vi "OP Model.vi"(8 "error in (no error)":errorcluster, 9 "Enum":enum16{"init", "Read", "Write"}(ring)=enum."Read", 10 "ArrayStr":string[](array[string]), 11 "Path":path) -> (0 "error out":errorcluster, 2 "ArrayStr out":string[](array[string]), 3 "Path out":path)   [LabVIEW 2014]
uses:
  <vilib>/Utility/xml.llb/Read From XML File(string).vi
  <vilib>/Utility/xml.llb/Write to XML File(string).vi
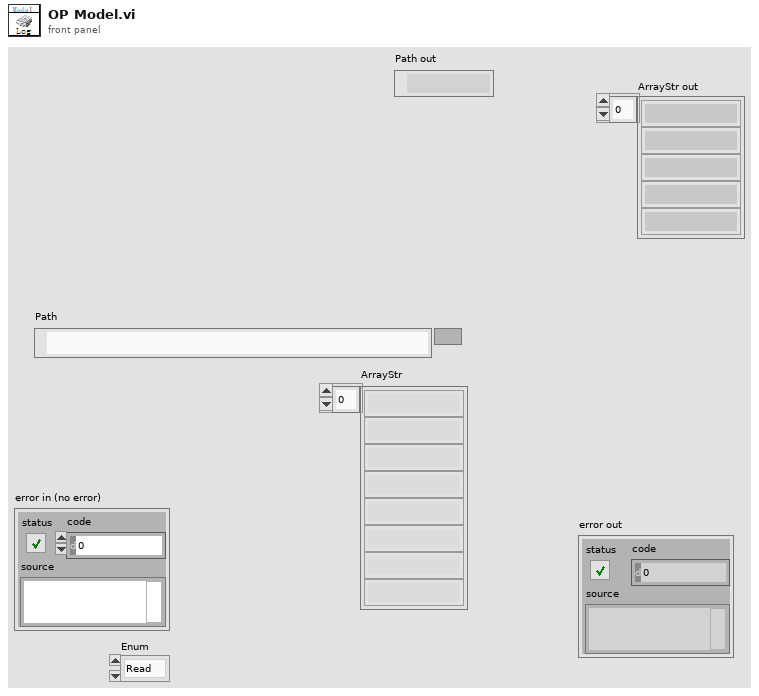
[diagram p1: front panel]
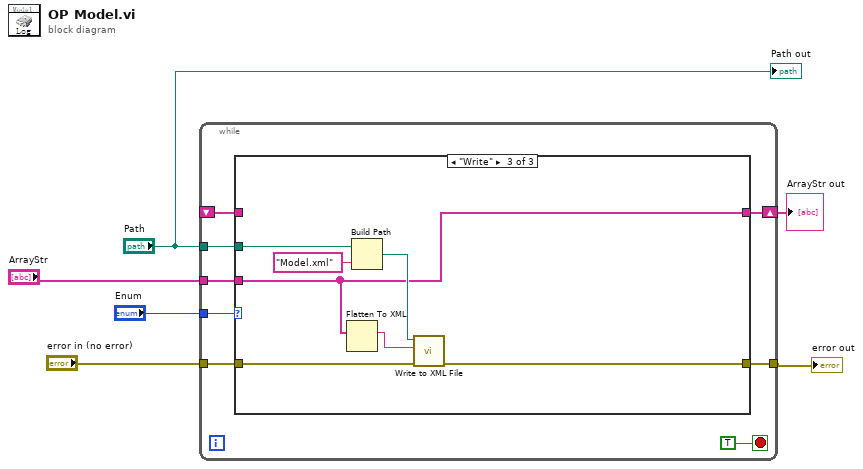
[diagram p0: block diagram]
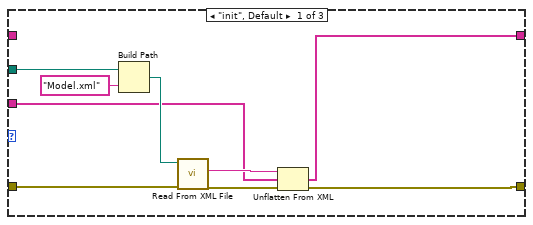
[diagram p2: hidden frame]
diagram:
  n1 = while {
    tunnel: "Enum" -> [w14]
    tunnel: "Path" -> [w13]
    tunnel: "error in (no error)" -> [w12]
    tunnel: "ArrayStr" -> [w11]
    shift-right: [w10] -> w1
    shift-left: _ -> [w8]
    tunnel: [w9] -> w3
    stop <- TRUE stop-if-true
    n2 = case shown="\"Write\"" w14 {
      tunnel: w13 -> [w22 _ w31]
      tunnel: w12 -> [w21 w24 w30]
      tunnel: w11 -> [w18 _ w27]
      tunnel: [w15 w25 w27] -> w10
      tunnel: [w16 w24 w29] -> w9
      tunnel: w8 -> [_ w25 _]
      frame "init", Default {
        n3 = Build Path(base path=w22, name or relative path="Model.xml") -> (appended path=w20:path)
        n4 = call-poly <vilib>:"Read From XML File.vi"("error in (no error)"=w21, "XML File Path"=w20) -> ("error out"=w17:errorcluster, "XML Elements"=w19:string)  [unwired: 7 in, 1 out]
        n5 = Unflatten From XML(xml string=w19, type=w18, error in (no error)=w17) -> (value=w15:string[], error out=w16:errorcluster)
      }
      frame "Read" {
      }
      frame "Write" {
        n6 = Flatten To XML(anything=w27) -> (xml string=w26:string)
        n7 = Build Path(base path=w31, name or relative path="Model.xml") -> (appended path=w28:path)
        n8 = call-poly <vilib>:"Write to XML File.vi"("error in (no error)"=w30, "XML Input"=w26, "XML File Path"=w28) -> ("error out"=w29:errorcluster)  [unwired: 6 in, 2 out]
      }
    }
  }
  "error out" <- w3
  "ArrayStr out" <- w1
  "Path out" <- "Path"
